vi "SP Read Array.vi"(8 "error in":errorcluster, 11 "Voltage Setpoint.lvclass":refnum<class "Voltage Setpoint.lvclass">) -> (0 "error out":errorcluster, 1 "Changed or First Call?":bool, 2 "Current Setpoint":dbl[](array[numeric]), 3 "Voltage Setpoint.lvclass 2":refnum<class "Voltage Setpoint.lvclass">)   [LabVIEW 2023, in "Voltage Setpoint.lvclass"]
uses:
  Voltage Setpoint.lvclass
  Voltage Setpoint.lvclass/Voltage Setpoint.ctl
  Parents/Setpoint/Setpoint.lvclass
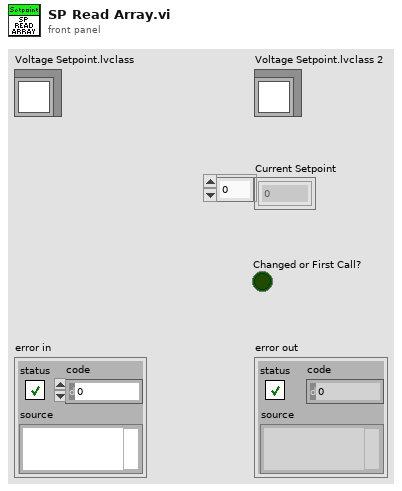
[diagram p1: front panel]
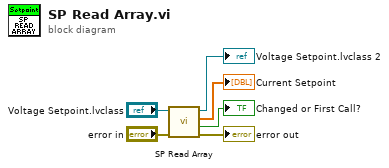
[diagram p0: block diagram]
diagram:
  n1 = call-parent "SP Read Array.vi"("error in"="error in", "Setpoint.lvclass"="Voltage Setpoint.lvclass") -> ("error out"=→"error out":errorcluster, "Changed or First Call?"=→"Changed or First Call?":bool, "Current Setpoint"=→"Current Setpoint":dbl[], "Setpoint.lvclass 2"=→"Voltage Setpoint.lvclass 2":refnum<class "Voltage Setpoint.lvclass">)  [unwired: 6 in]
